vi "LS One Hour Data Loop.vi"(11 "FPGA OneHour Ref":T1) -> ()   [LabVIEW 2013]
uses:
  Controls/FPGA_OneHour_Reference.ctl
  <vilib>/rvi/interface/common/niFpgaWaitOnOcc.vi
  <vilib>/Utility/error.llb/Error Cluster From Error Code.vi
  <vilib>/rvi/errors/niLvFpgaAdjustHostInterfaceError.vi
  <vilib>/rvi/interface/nirviMethod/nirviMethod.xnode
  FPGA Bitfiles/LSDurabilityMain_Alternate.lvbitx
  <vilib>/rvi/interface/nirviReadWriteControl/nirviReadWriteControl.xnode
  <vilib>/FPGAPlugInAG/sbRIO-9626/niLvFpga_ReadFifo_sbRIO-9626.vi
  <vilib>/rvi/errors/niLvFpgaMergeErrorWithErrorCode.vi
  NiFpgaLv.dll
panel:
  in  "LoopWait(ms)":u32=100
  in  "Sections":i32=100
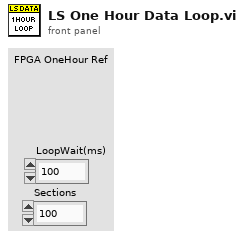
[diagram p1: front panel]
types:
  T1 = typedef "FPGA_OneHour_Reference.ctl" = refnum<k20>
  T2 = cluster{"FPGA OneHour Ref":T1, "Time":dbl, "PtsTaken":i32, "Pts/File":i32, "10AveWait":u32, "Stored Filepath":path, "FileIndex":i32, "FilesUsed":i32}
  T3 = enum16{"open", "replace", "create", "open or create", "replace or create", "replace or create with confirmation"}
  T4 = cluster{"Running?":bool, "Profile Record":bool, "RecordInterval":i32, "RecordDuration":i32, "RecordFreq":i32, "Data Filepath":path, "Hr Record":bool, "Serial Numbers":string[]}
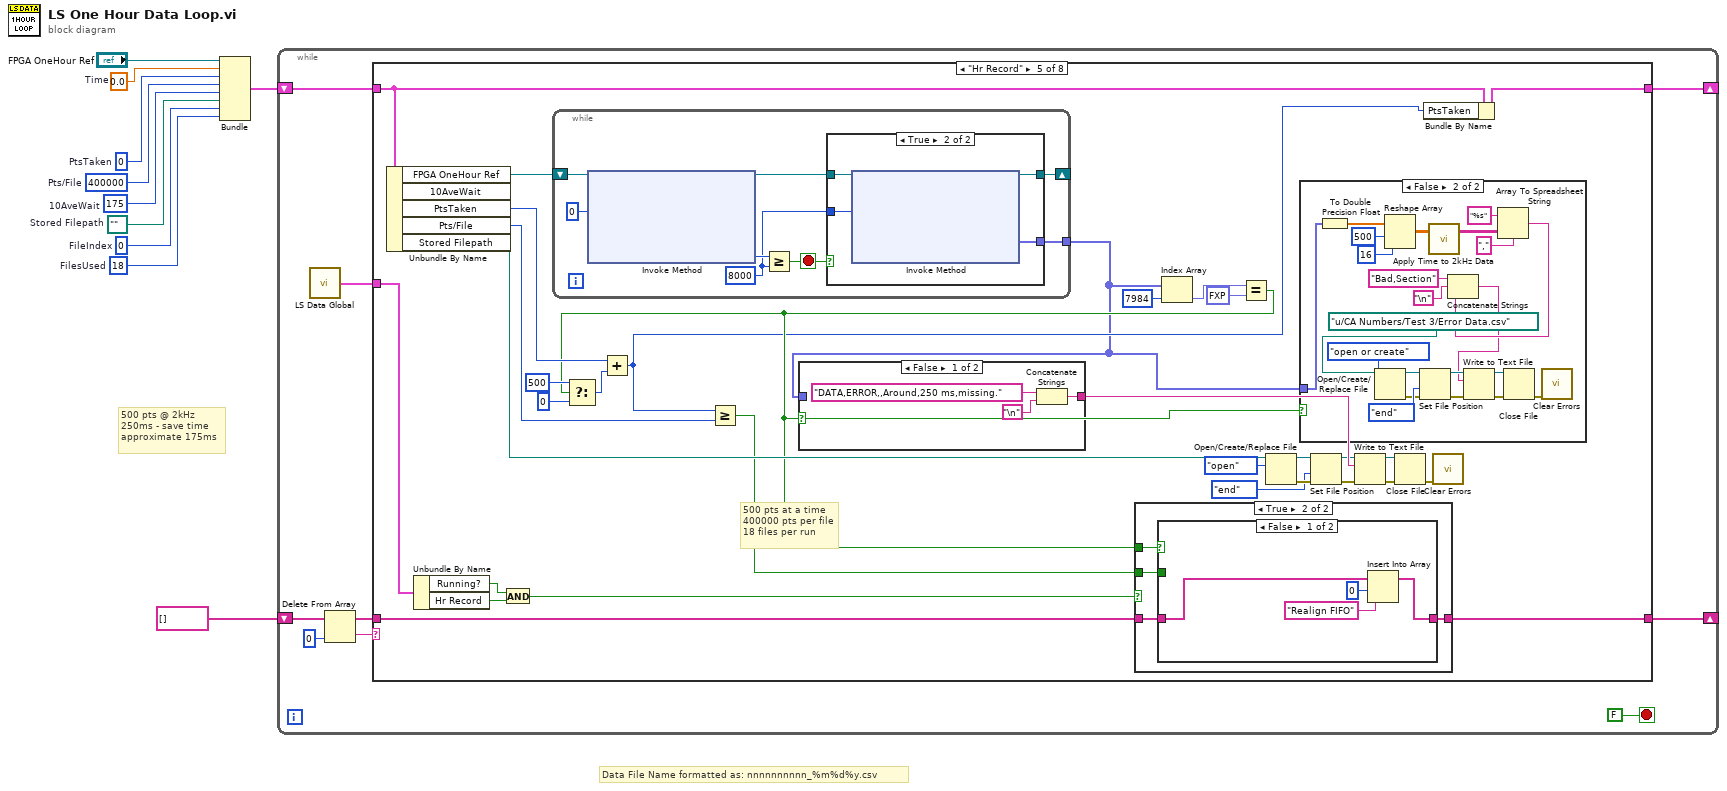
[diagram p0: block diagram]
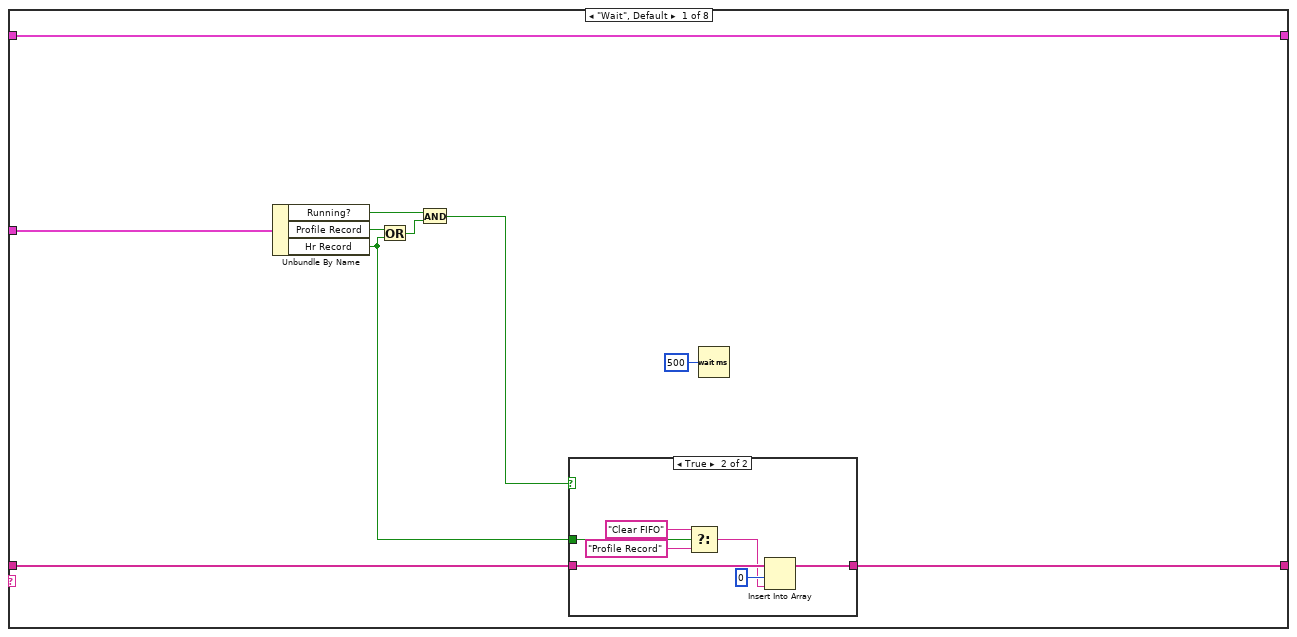
[diagram p2: hidden frame]
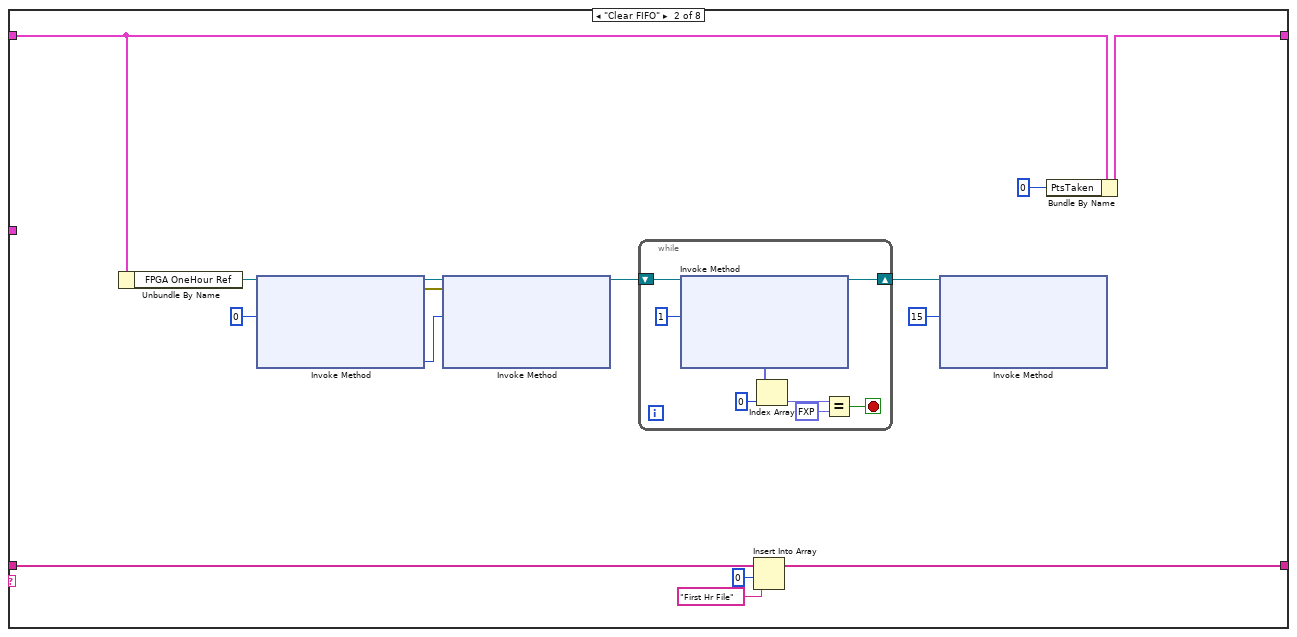
[diagram p4: hidden frame]
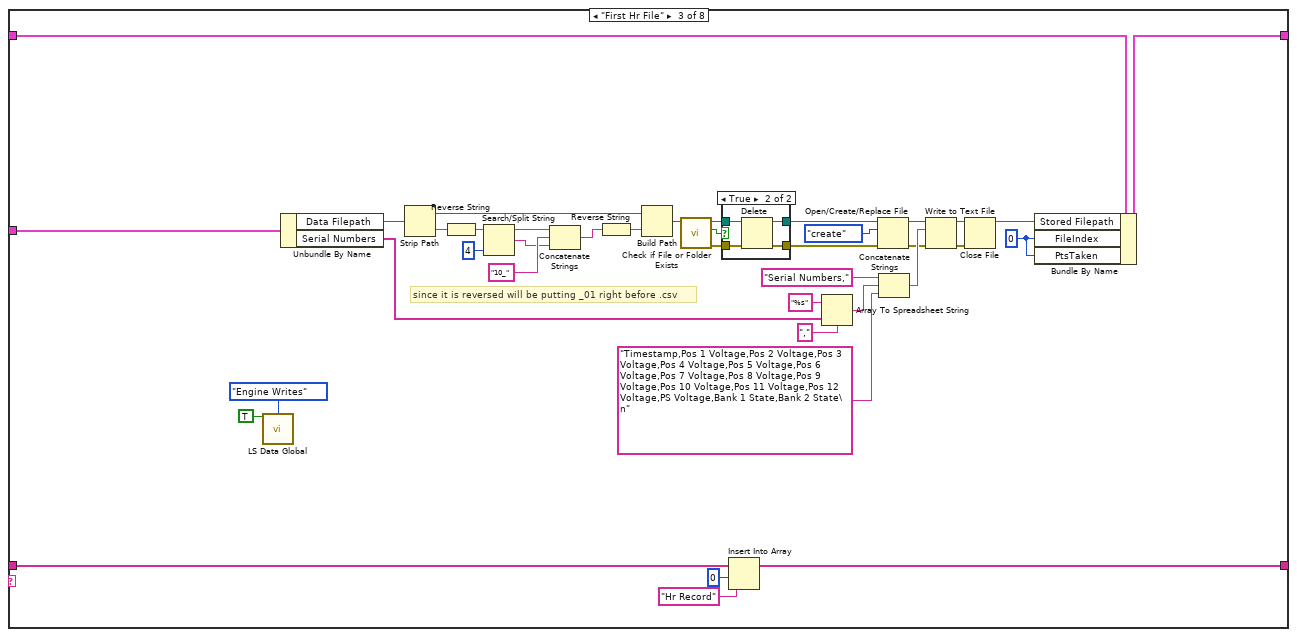
[diagram p5: hidden frame]
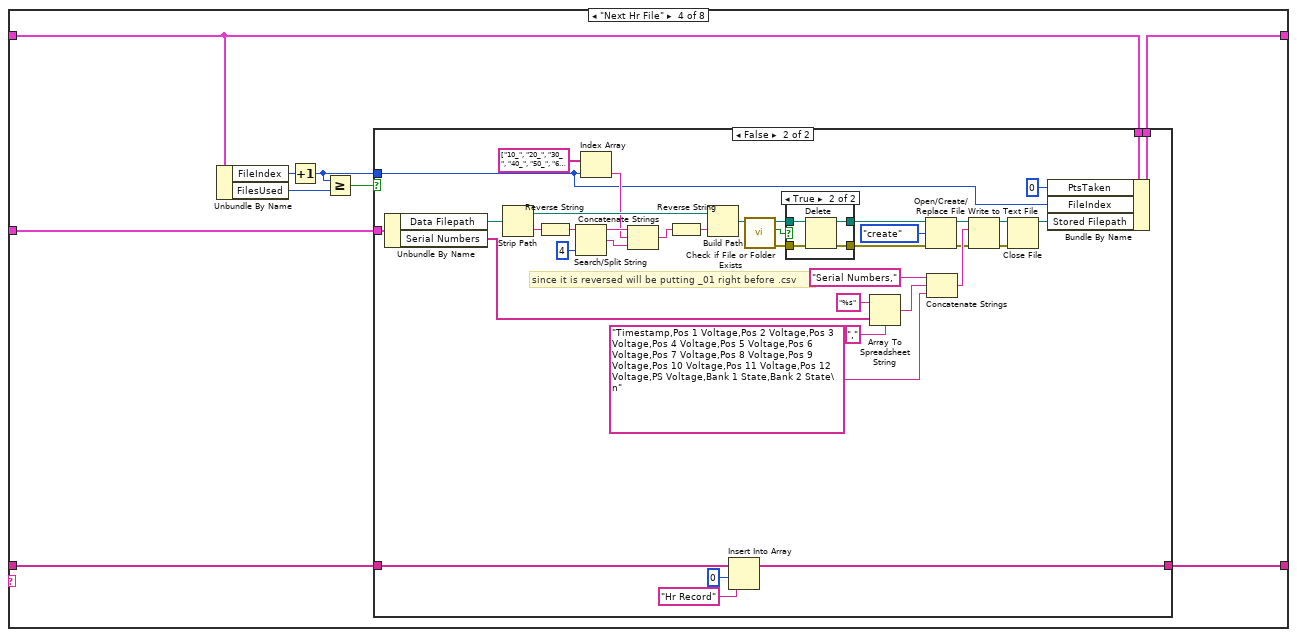
[diagram p7: hidden frame]
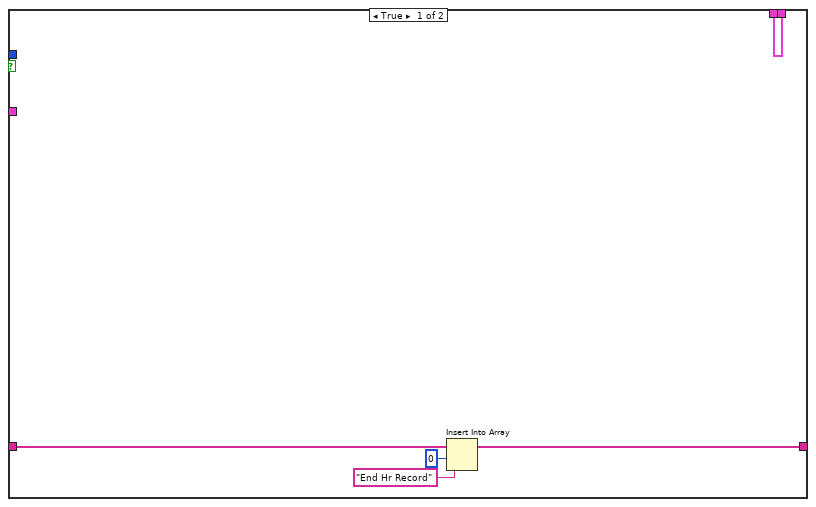
[diagram p8: hidden frame]
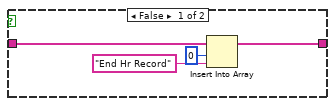
[diagram p11: hidden frame]
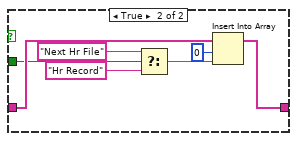
[diagram p12: hidden frame]
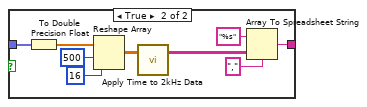
[diagram p13: hidden frame]
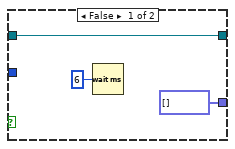
[diagram p14: hidden frame]
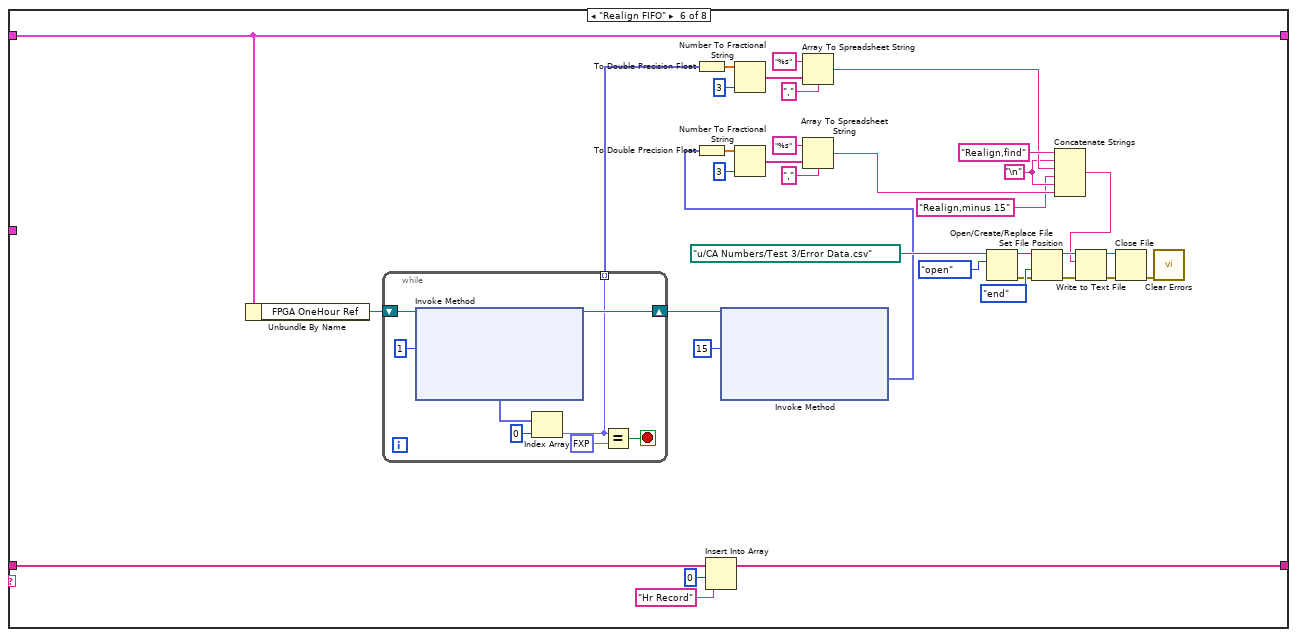
[diagram p15: hidden frame]
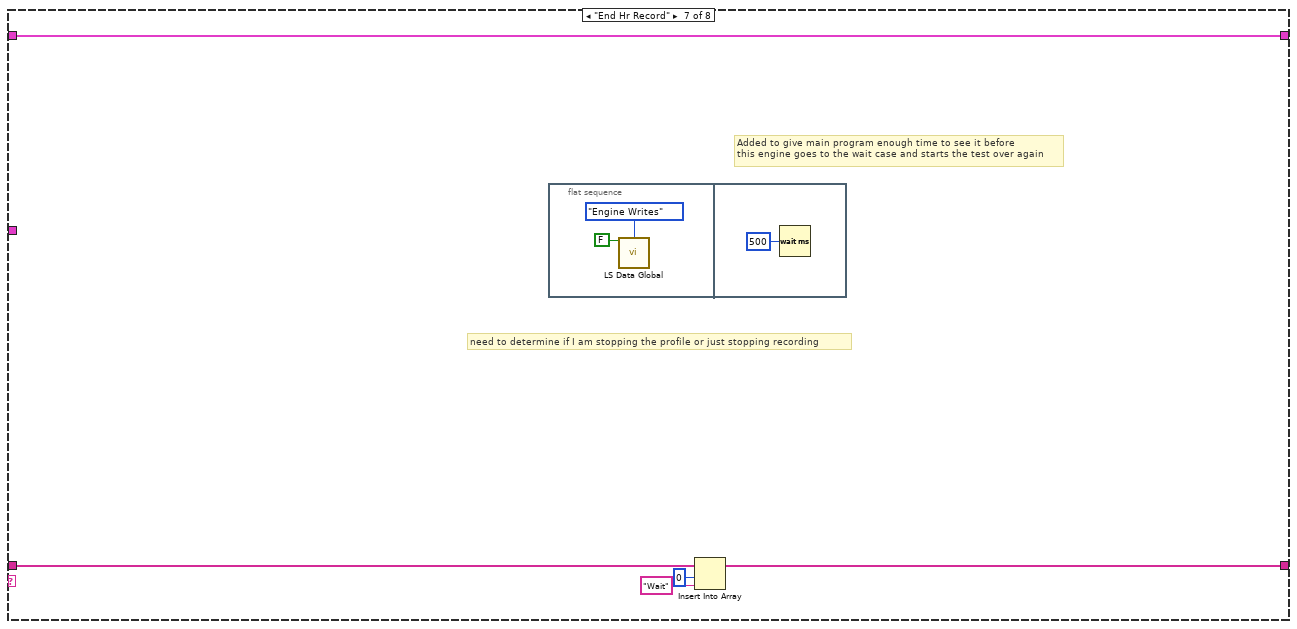
[diagram p16: hidden frame]
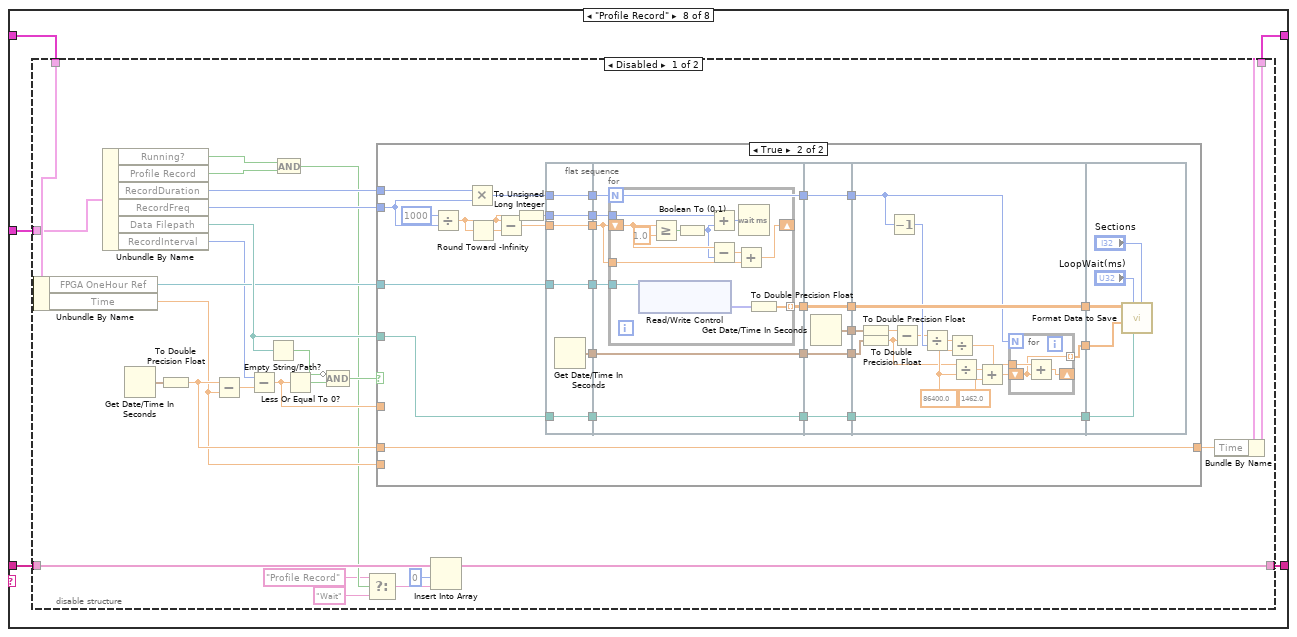
[diagram p17: hidden frame]
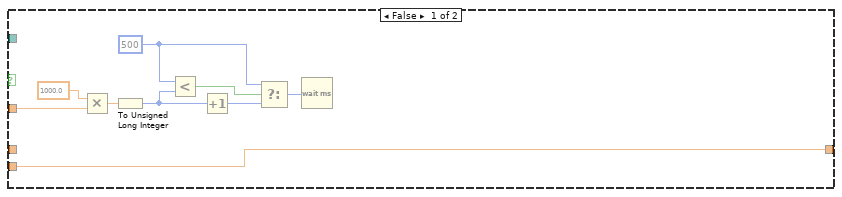
[diagram p18: hidden frame]
diagram:
  w1 = 18  # FilesUsed
  w2 = 400000  # Pts/File
  w4 = 0  # FileIndex
  w5 = path ""  # Stored Filepath
  w6 = u32 175  # 10AveWait
  w7 = 0  # PtsTaken
  w10 = 0.0  # Time
  # "500 pts @ 2kHz\n250ms - save time\napproximate 175ms"
  # "Data File Name formatted as: nnnnnnnnnn_%m%d%y.csv"
  n1 = Bundle("FPGA OneHour Ref"="FPGA OneHour Ref", "Time"=w10, "PtsTaken"=w7, "Pts/File"=w2, "10AveWait"=w6, "Stored Filepath"=w5, "FileIndex"=w4, "FilesUsed"=w1) -> (w9:T2)  [unwired: 1 in]
  n2 = while {
    shift-right: [w17] -> _
    shift-left: w9 -> [w18]
    shift-right: [w14] -> _
    shift-left: string[] [] -> [w16]
    stop <- FALSE stop-if-true
    n3 = call "LS Data Global.vi"() -> ("LS Cluster Out"=w15:T4)  [unwired: 14 in, 1 out]
    n4 = Delete From Array(array=w16, index=0) -> (deleted portion=w12:string, array with subset deleted=w11:string[])  [unwired: 1 in]
    n5 = case shown="\"Hr Record\"" w12 {
      tunnel: w11 -> [w26 w47 w86 w106 w177 w294 w312 w318]
      tunnel: [w25 w45 w85 w112 w178 w293 w311 w317] -> w14
      tunnel: w15 -> [w27 _ w98 w114 w194 _ _ w319]
      tunnel: w18 -> [w24 w43 w99 w111 w172 w297 w313 w321]
      tunnel: [w24 w42 w97 w113 w171 w297 w313 w320] -> w17
      frame "Wait", Default {
        n6 = Unbundle By Name(w27) -> ("Running?"=w28:bool, "Profile Record"=w23:bool, "Hr Record"=w21:bool)
        n7 = Or(x=w23, y=w21) -> (x .or. y?=w22:bool)
        n8 = And(x=w28, y=w22) -> (x .and. y?=w20:bool)
        n9 = case shown="True" w20 {
          tunnel: w26 -> [w30 w37]
          tunnel: [w30 w36] -> w25
          tunnel: w21 -> [_ w34]
          frame False {
          }
          frame True {
            n10 = Select(t="Clear FIFO" ("new element/subarray"), s=w34, f="Profile Record" ("new element/subarray")) -> (s? t:f=w32:string)
            n11 = Insert Into Array(array=w37, index=0, new element=w32) -> (w36:string[])
          }
        }
        n12 = Wait (ms)(milliseconds to wait=u32 500) -> ()  [unwired: 1 out]
      }
      frame "Clear FIFO" {
        n13 = Unbundle By Name(w43) -> ("FPGA OneHour Ref"=w52:T1)
        n14 = xnode "Invoke Method"("FPGA VI Reference In"=w52, "Number of Elements"=u32 0) -> ("FPGA VI Reference Out"=w51:T1, "error out"=w50:errorcluster, "Elements Remaining"=w48:u32)  [unwired: 2 in, 1 out]
        n15 = xnode "Invoke Method"("FPGA VI Reference In"=w51, "error in"=w50, "Number of Elements"=w48) -> ("FPGA VI Reference Out"=w40:T1)  [unwired: 1 in, 3 out]
        n16 = while {
          shift-right: [w59] -> w38
          shift-left: w40 -> [w60]
          stop <- w53 stop-if-true
          n17 = xnode "Invoke Method"("FPGA VI Reference In"=w60, "Number of Elements"=u32 1) -> ("FPGA VI Reference Out"=w59:T1, "Data"=w57:fxp<+/-,18,5>[])  [unwired: 2 in, 2 out]
          n18 = Index Array(array=w57, index=0) -> (element=w55:fxp<+/-,18,5>)
          n19 = Equal?(x=w55, y=fxp<+/-,18,5> -15.0 ("lower limit")) -> (x = y?=w53:bool)
        }
        n20 = Insert Into Array(array=w47, index=0, new element="First Hr File" ("new element/subarray")) -> (w45:string[])
        n21 = xnode "Invoke Method"("FPGA VI Reference In"=w38, "Number of Elements"=u32 15) -> ()  [unwired: 2 in, 4 out]
        n22 = Bundle By Name(cluster=w43, "PtsTaken"=0) -> (w42:T2)
      }
      frame "First Hr File" {
        w63 = 0 ("FileIndex")
        # "since it is reversed will be putting _01 right before .csv"
        n23 = call "LS Data Global.vi"("Recording In"=TRUE, "Mode"=enum16{"Read", "Engine Writes", "Main Writes"}."Engine Writes") -> ()  [unwired: 12 in, 2 out]
        n24 = Unbundle By Name(w98) -> ("Data Filepath"=w96:path, "Serial Numbers"=w64:string[])
        n25 = Strip Path(path=w96) -> (stripped path=w95:path, name=w94:string)
        n26 = Reverse String(1:w94) -> (0:w92:string)
        n27 = Search/Split String(string=w92, offset (0)=4) -> (substring before match=w90:string, match + rest of string=w87:string)  [unwired: 1 in, 1 out]
        n28 = Concatenate Strings(w90, "10_", w87) -> (w89:string)
        n29 = Reverse String(1:w89) -> (0:w93:string)
        n30 = Build Path(base path=w95, name or relative path=w93) -> (appended path=w82:path)
        n31 = call <vilib>:"Check if File or Folder Exists.vi"("path"=w82) -> ("error out"=w67:errorcluster, "file or folder exists?"=w81:bool, "dup path"=w80:path)  [unwired: 8 in]
        n32 = case shown="True" w81 {
          tunnel: w80 -> [w101 w105]
          tunnel: [w101 w104] -> w69
          tunnel: w67 -> [w100 w103]
          tunnel: [w100 w102] -> w66
          frame False {
          }
          frame True {
            n33 = Delete(path (use dialog)=w105, error in=w103) -> (deleted path=w104:path, error out=w102:errorcluster)  [unwired: 3 in, 1 out]
          }
        }
        n34 = Insert Into Array(array=w86, index=0, new element="Hr Record" ("new element/subarray")) -> (w85:string[])
        n35 = Array To Spreadsheet String(delimiter (Tab)=",", array=w64, 3:"%s" ("format string")) -> (spreadsheet string=w79:string)
        n36 = Open/Create/Replace File(file path (use dialog)=w69, error in=w66, operation (0:open)=T3."create") -> (refnum out=w73:refnum<file>, error out=w71:errorcluster)  [unwired: 3 in, 1 out]
        n37 = Concatenate Strings("Serial Numbers," ("string"), w79, "Timestamp,Pos 1 Voltage,Pos 2 Voltage,Pos 3 Voltage,Pos 4 Voltage,Pos 5 Voltage,Pos 6 Voltage,Pos 7 Voltage,Pos 8 Voltage,Pos 9 Voltage,Pos 10 Voltage,Pos 11 Voltage,Pos 12 Voltage,PS Voltage,Bank 1 State,Bank 2 State\n") -> (w76:string)
        n38 = Write to Text File(file (use dialog)=w73, text=w76, error in=w71) -> (refnum out=w74:refnum<file>, error out=w72:errorcluster)  [unwired: 1 in, 1 out]
        n39 = Close File(refnum=w74, error in=w72) -> (path=w68:path)  [unwired: 1 out]
        n40 = Bundle By Name(cluster=w99, "Stored Filepath"=w68, "FileIndex"=w63, "PtsTaken"=w63) -> (w97:T2)
      }
      frame "Next Hr File" {
        n41 = Unbundle By Name(w111) -> ("FileIndex"=w110:i32, "FilesUsed"=w109:i32)
        n42 = Increment(x=w110) -> (x+1=w108:i32)
        n43 = Greater Or Equal?(x=w108, y=w109) -> (x >= y?=w107:bool)
        n44 = case shown="False" w107 {
          tunnel: w114 -> [_ w158]
          tunnel: [w119 w157] -> w113
          tunnel: [w117 w146] -> w112
          tunnel: w111 -> [w119 w124]
          tunnel: w108 -> [_ w121]
          tunnel: w106 -> [w118 w147]
          frame True {
            n45 = Insert Into Array(array=w118, index=0, new element="End Hr Record" ("new element/subarray")) -> (w117:string[])
          }
          frame False {
            # "since it is reversed will be putting _01 right before .csv"
            n46 = Unbundle By Name(w158) -> ("Data Filepath"=w156:path, "Serial Numbers"=w125:string[])
            n47 = Strip Path(path=w156) -> (stripped path=w155:path, name=w154:string)
            n48 = Reverse String(1:w154) -> (0:w152:string)
            n49 = Search/Split String(string=w152, offset (0)=4) -> (substring before match=w150:string, match + rest of string=w148:string)  [unwired: 1 in, 1 out]
            n50 = Index Array(array=string[] ["10_", "20_", "30_", "40_", "50_", "60_", "70_", "80_", "90_", "01_", "11_", "21_", "31_", "41_", "51_", "61_", "71_", "81_", "91_", "02_", "12_", "22_", "32_", "42_", "52_", "62_", "72_", "82_", "92_", "03_", "13_", "23_"], index=w121) -> (element=w122:string)
            n51 = Concatenate Strings(w150, w122, w148) -> (w149:string)
            n52 = Reverse String(1:w149) -> (0:w153:string)
            n53 = Build Path(base path=w155, name or relative path=w153) -> (appended path=w143:path)
            n54 = Insert Into Array(array=w147, index=0, new element="Hr Record" ("new element/subarray")) -> (w146:string[])
            n55 = call <vilib>:"Check if File or Folder Exists.vi"("path"=w143) -> ("error out"=w128:errorcluster, "file or folder exists?"=w142:bool, "dup path"=w141:path)  [unwired: 8 in]
            n56 = case shown="True" w142 {
              tunnel: w141 -> [w160 w164]
              tunnel: [w160 w163] -> w130
              tunnel: w128 -> [w159 w162]
              tunnel: [w159 w161] -> w127
              frame False {
              }
              frame True {
                n57 = Delete(path (use dialog)=w164, error in=w162) -> (deleted path=w163:path, error out=w161:errorcluster)  [unwired: 3 in, 1 out]
              }
            }
            n58 = Array To Spreadsheet String(delimiter (Tab)=",", array=w125, 3:"%s" ("format string")) -> (spreadsheet string=w140:string)
            n59 = Open/Create/Replace File(file path (use dialog)=w130, error in=w127, operation (0:open)=T3."create") -> (refnum out=w134:refnum<file>, error out=w132:errorcluster)  [unwired: 3 in, 1 out]
            n60 = Concatenate Strings("Serial Numbers," ("string"), w140, "Timestamp,Pos 1 Voltage,Pos 2 Voltage,Pos 3 Voltage,Pos 4 Voltage,Pos 5 Voltage,Pos 6 Voltage,Pos 7 Voltage,Pos 8 Voltage,Pos 9 Voltage,Pos 10 Voltage,Pos 11 Voltage,Pos 12 Voltage,PS Voltage,Bank 1 State,Bank 2 State\n") -> (w137:string)
            n61 = Write to Text File(file (use dialog)=w134, text=w137, error in=w132) -> (refnum out=w135:refnum<file>, error out=w133:errorcluster)  [unwired: 1 in, 1 out]
            n62 = Close File(refnum=w135, error in=w133) -> (path=w129:path)  [unwired: 1 out]
            n63 = Bundle By Name(cluster=w124, "PtsTaken"=0, "FileIndex"=w121, "Stored Filepath"=w129) -> (w157:T2)
          }
        }
      }
      frame "Hr Record" {
        # "500 pts at a time\n400000 pts per file\n18 files per run"
        n64 = Unbundle By Name(w172) -> ("FPGA OneHour Ref"=w166:T1, "PtsTaken"=w176:i32, "Pts/File"=w170:i32, "Stored Filepath"=w183:path)  [unwired: 1 out]
        n65 = Unbundle By Name(w194) -> ("Running?"=w195:bool, "Hr Record"=w196:bool)
        n66 = And(x=w195, y=w196) -> (x .and. y?=w179:bool)
        n67 = while {
          shift-right: [w252] -> _
          shift-left: w166 -> [w255]
          tunnel: [w251] -> w165
          stop <- w250 stop-if-true
          w254 = u32 8000 ("y")
          n68 = xnode "Invoke Method"("FPGA VI Reference In"=w255, "Number of Elements"=u32 0) -> ("FPGA VI Reference Out"=w253:T1, "Elements Remaining"=w256:u32)  [unwired: 2 in, 2 out]
          n69 = Greater Or Equal?(x=w256, y=w254) -> (x >= y?=w250:bool)
          n70 = case shown="True" w250 {
            tunnel: w254 -> [_ w264]
            tunnel: w253 -> [w260 w263]
            tunnel: [w260 w262] -> w252
            tunnel: [fxp<+/-,18,5>[] [] ("Data") w261] -> w251
            frame False {
              n71 = Wait (ms)(milliseconds to wait=u32 6) -> ()  [unwired: 1 out]
            }
            frame True {
              n72 = xnode "Invoke Method"("FPGA VI Reference In"=w263, "Number of Elements"=w264) -> ("FPGA VI Reference Out"=w262:T1, "Data"=w261:fxp<+/-,18,5>[])  [unwired: 2 in, 2 out]
            }
          }
        }
        n73 = Index Array(array=w165, index=7984) -> (element=w181:fxp<+/-,18,5>)
        n74 = Equal?(x=w181, y=fxp<+/-,18,5> -15.0) -> (x = y?=w168:bool)
        n75 = Select(t=500 ("PtsTaken"), s=w168, f=0 ("PtsTaken")) -> (s? t:f=w173:i32)
        n76 = Add(x=w176, y=w173) -> (x+y=w167:i32)
        n77 = Greater Or Equal?(x=w167, y=w170) -> (x >= y?=w169:bool)
        n78 = case shown="False" w168 {
          tunnel: [w238 w244] -> w186
          tunnel: w165 -> [_ w243]
          frame False {
            n79 = Concatenate Strings("DATA,ERROR,,Around,250 ms,missing." ("string"), "\n") -> (w238:string)
          }
          frame True {
            n80 = To Double Precision Float(number=w243) -> (double precision float=w247:dbl[])
            n81 = Reshape Array(w247, 500 ("dimension size"), 16 ("dimension size")) -> (w242:dbl[][])
            n82 = call "Apply Time to 2kHz Data.vi"("Data In"=w242) -> ("Data Out"=w241:string[][])  [unwired: 2 in]
            n83 = Array To Spreadsheet String(delimiter (Tab)=",", array=w241, 3:"%s" ("format string")) -> (spreadsheet string=w244:string)
          }
        }
        n84 = case shown="True" w179 {
          tunnel: w177 -> [w221 w225]
          tunnel: [w220 w224] -> w178
          tunnel: w168 -> [_ w226]
          tunnel: w169 -> [_ w223]
          frame False {
            n85 = Insert Into Array(array=w221, index=0, new element="End Hr Record") -> (w220:string[])
          }
          frame True {
            n86 = case shown="False" w226 {
              tunnel: w225 -> [w230 w237]
              tunnel: [w229 w236] -> w224
              tunnel: w223 -> [_ w234]
              frame False {
                n87 = Insert Into Array(array=w230, index=0, new element="Realign FIFO" ("new element/subarray")) -> (w229:string[])
              }
              frame True {
                n88 = Select(t="Next Hr File", s=w234, f="Hr Record") -> (s? t:f=w233:string)
                n89 = Insert Into Array(array=w237, index=0, new element=w233) -> (w236:string[])
              }
            }
          }
        }
        n90 = Open/Create/Replace File(file path (use dialog)=w183, operation (0:open)=T3."open") -> (refnum out=w189:refnum<file>, error out=w188:errorcluster)  [unwired: 4 in, 1 out]
        n91 = case shown="False" w168 {
          tunnel: w165 -> [_ w213]
          frame True {
          }
          frame False {
            n92 = To Double Precision Float(number=w213) -> (double precision float=w216:dbl[])
            n93 = Open/Create/Replace File(file path (use dialog)=path "u:/CA Numbers/Test 3/Error Data.csv" ("base path"), operation (0:open)=T3."open or create") -> (refnum out=w206:refnum<file>, error out=w207:errorcluster)  [unwired: 4 in, 1 out]
            n94 = Reshape Array(w216, 500 ("dimension size"), 16 ("dimension size")) -> (w212:dbl[][])
            n95 = Set File Position(refnum=w206, from (0:start)=enum16{"start", "end", "current"}."end", error in=w207) -> (refnum out=w209:refnum<file>, error out=w210:errorcluster)  [unwired: 1 in]
            n96 = call "Apply Time to 2kHz Data.vi"("Data In"=w212) -> ("Data Out"=w211:string[][])  [unwired: 2 in]
            n97 = Array To Spreadsheet String(delimiter (Tab)=",", array=w211, 3:"%s" ("format string")) -> (spreadsheet string=w199:string)
            n98 = Concatenate Strings("Bad,Section" ("string"), "\n", w199) -> (w198:string)
            n99 = Write to Text File(file (use dialog)=w209, text=w198, error in=w210) -> (refnum out=w203:refnum<file>, error out=w202:errorcluster)  [unwired: 1 in, 1 out]
            n100 = Close File(refnum=w203, error in=w202) -> (error out=w204:errorcluster)  [unwired: 1 out]
            n101 = call <vilib>:"Clear Errors.vi"("error in (no error)"=w204) -> ()  [unwired: 6 in, 1 out]
          }
        }
        n102 = Set File Position(refnum=w189, from (0:start)=enum16{"start", "end", "current"}."end", error in=w188) -> (refnum out=w185:refnum<file>, error out=w184:errorcluster)  [unwired: 1 in]
        n103 = Write to Text File(file (use dialog)=w185, text=w186, error in=w184) -> (refnum out=w192:refnum<file>, error out=w193:errorcluster)  [unwired: 1 in, 1 out]
        n104 = Close File(refnum=w192, error in=w193) -> (error out=w191:errorcluster)  [unwired: 1 out]
        n105 = Bundle By Name(cluster=w172, "PtsTaken"=w167) -> (w171:T2)
        n106 = call <vilib>:"Clear Errors.vi"("error in (no error)"=w191) -> ()  [unwired: 6 in, 1 out]
      }
      frame "Realign FIFO" {
        w273 = "\n"
        n107 = Unbundle By Name(w297) -> ("FPGA OneHour Ref"=w300:T1)
        n108 = while {
          shift-right: [w307] -> w298
          shift-left: w300 -> [w308]
          tunnel: [w301] -> w277 mode=indexing
          stop <- w302 stop-if-true
          n109 = xnode "Invoke Method"("FPGA VI Reference In"=w308, "Number of Elements"=u32 1) -> ("FPGA VI Reference Out"=w307:T1, "Data"=w305:fxp<+/-,18,5>[])  [unwired: 2 in, 2 out]
          n110 = Index Array(array=w305, index=0) -> (element=w301:fxp<+/-,18,5>)
          n111 = Equal?(x=w301, y=fxp<+/-,18,5> -15.0 ("lower limit")) -> (x = y?=w302:bool)
        }
        n112 = To Double Precision Float(number=w277) -> (double precision float=w275:dbl[])
        n113 = Insert Into Array(array=w294, index=0, new element="Hr Record" ("new element/subarray")) -> (w293:string[])
        n114 = xnode "Invoke Method"("FPGA VI Reference In"=w298, "Number of Elements"=u32 15) -> ("Data"=w267:fxp<+/-,18,5>[])  [unwired: 2 in, 3 out]
        n115 = To Double Precision Float(number=w267) -> (double precision float=w271:dbl[])
        n116 = Number To Fractional String(number=w275, precision (6)=i16 3) -> (F-format string=w274:string[])  [unwired: 2 in]
        n117 = Number To Fractional String(number=w271, precision (6)=i16 3) -> (F-format string=w272:string[])  [unwired: 2 in]
        n118 = Array To Spreadsheet String(delimiter (Tab)=",", array=w274, 3:"%s" ("format string")) -> (spreadsheet string=w280:string)
        n119 = Array To Spreadsheet String(delimiter (Tab)=",", array=w272, 3:"%s" ("format string")) -> (spreadsheet string=w266:string)
        n120 = Open/Create/Replace File(file path (use dialog)=path "u:/CA Numbers/Test 3/Error Data.csv" ("base path"), operation (0:open)=T3."open") -> (refnum out=w286:refnum<file>, error out=w287:errorcluster)  [unwired: 4 in, 1 out]
        n121 = Set File Position(refnum=w286, from (0:start)=enum16{"start", "end", "current"}."end", error in=w287) -> (refnum out=w289:refnum<file>, error out=w290:errorcluster)  [unwired: 1 in]
        n122 = Concatenate Strings("Realign,find" ("string"), w273, w280, "Realign,minus 15" ("string"), w273, w266) -> (w279:string)
        n123 = Write to Text File(file (use dialog)=w289, text=w279, error in=w290) -> (refnum out=w283:refnum<file>, error out=w282:errorcluster)  [unwired: 1 in, 1 out]
        n124 = Close File(refnum=w283, error in=w282) -> (error out=w284:errorcluster)  [unwired: 1 out]
        n125 = call <vilib>:"Clear Errors.vi"("error in (no error)"=w284) -> ()  [unwired: 6 in, 1 out]
      }
      frame "End Hr Record" {
        # "Added to give main program enough time to see it before\nthis engine goes to the wait case and starts the test over again"
        # "need to determine if I am stopping the profile or just stopping recording"
        n126 = flat-sequence {
          frame #0 {
            n127 = call "LS Data Global.vi"("Recording In"=FALSE, "Mode"=enum16{"Read", "Engine Writes", "Main Writes"}."Engine Writes") -> ()  [unwired: 12 in, 2 out]
          }
          frame #1 {
            n128 = Wait (ms)(milliseconds to wait=u32 500) -> ()  [unwired: 1 out]
          }
        }
        n129 = Insert Into Array(array=w312, index=0, new element="Wait" ("new element/subarray")) -> (w311:string[])
      }
      frame "Profile Record" {
        n130 = disable-structure shown="Disabled" {
          disable-tunnel: w321 -> [w347 w441]
          disable-tunnel: [w346 w441] -> w320
          disable-tunnel: w319 -> [w345 _]
          disable-tunnel: w318 -> [w328 w440]
          disable-tunnel: [w327 w440] -> w317
          frame Disabled {
            n131 = Unbundle By Name(w347) -> ("FPGA OneHour Ref"=w339:T1, "Time"=w333:dbl)
            n132 = Unbundle By Name(w345) -> ("Running?"=w330:bool, "Profile Record"=w329:bool, "RecordDuration"=w342:i32, "RecordFreq"=w343:i32, "Data Filepath"=w344:path, "RecordInterval"=w331:i32)
            n133 = Get Date/Time In Seconds() -> (seconds since 1Jan1904=w341:timestamp)
            n134 = To Double Precision Float(number=w341) -> (double precision float=w334:dbl)
            n135 = Subtract(x=w334, y=w333) -> (x-y=w338:dbl)
            n136 = Subtract(x=w331, y=w338) -> (x-y=w332:dbl)
            n137 = Empty String/Path?(string/path=w344) -> (empty?=w336:bool)
            n138 = And(x=w330, y=w329) -> (x .and. y?=w325:bool)
            n139 = Less Or Equal To 0?(x=w332) -> (x <= 0?=w337:bool)
            n140 = Compound Arithmetic op=AND(invert w336, w337) -> (w335:bool)
            n141 = Select(t="Profile Record", s=w325, f="Wait") -> (s? t:f=w322:string)
            n142 = case shown="True" w335 {
              tunnel: w343 -> [_ w378]
              tunnel: w342 -> [_ w384]
              tunnel: w339 -> [_ w381]
              tunnel: w334 -> [_ w380]
              tunnel: [w356 w380] -> w340
              tunnel: w333 -> [w356 _]
              tunnel: w332 -> [w350 _]
              tunnel: w344 -> [_ w357]
              frame False {
                w355 = u32 500 ("milliseconds to wait")
                n143 = Multiply(x=1000.0 ("y"), y=w350) -> (x*y=w352:dbl)
                n144 = To Unsigned Long Integer(number=w352) -> (unsigned 32bit integer=w349:u32)
                n145 = Less?(x=w355, y=w349) -> (x < y?=w353:bool)
                n146 = Increment(x=w349) -> (x+1=w348:u32)
                n147 = Select(t=w355, s=w353, f=w348) -> (s? t:f=w354:u32)
                n148 = Wait (ms)(milliseconds to wait=w354) -> ()  [unwired: 1 out]
              }
              frame True {
                n149 = Divide(x=1000, y=w378) -> (x/y=w383:dbl)
                n150 = Multiply(x=w384, y=w378) -> (x*y=w371:i32)
                n151 = Round Toward -Infinity(1:w383) -> (0:w385:dbl)
                n152 = Subtract(x=w383, y=w385) -> (x-y=w377:dbl)
                n153 = To Unsigned Long Integer(number=w383) -> (unsigned 32bit integer=w382:u32)
                n154 = flat-sequence {
                  tunnel: w377 -> [w388]
                  tunnel: w381 -> [w389]
                  tunnel: w382 -> [w390]
                  tunnel: w371 -> [w391]
                  tunnel: [w391] -> w376
                  tunnel: [w390] -> w375
                  tunnel: [w389] -> w374
                  tunnel: [w388] -> w373
                  tunnel: [w387] -> w366
                  tunnel: [w386] -> w358
                  tunnel: w357 -> [w386]
                  tunnel: w376 -> [w394]
                  tunnel: w375 -> [w398]
                  tunnel: w374 -> [w397]
                  tunnel: w373 -> [w392]
                  tunnel: [w396] -> w372
                  tunnel: [w395] -> w367
                  tunnel: w366 -> [w395]
                  tunnel: [w394] -> w364
                  tunnel: [w393] -> w359
                  tunnel: w358 -> [w393]
                  tunnel: w372 -> [w415]
                  tunnel: [w415] -> w370
                  tunnel: [w414] -> w369
                  tunnel: [w413] -> w368
                  tunnel: w367 -> [w413]
                  tunnel: [w412] -> w365
                  tunnel: w364 -> [w412]
                  tunnel: [w411] -> w360
                  tunnel: w359 -> [w411]
                  tunnel: w370 -> [w431]
                  tunnel: w369 -> [w425]
                  tunnel: w368 -> [w424]
                  tunnel: w365 -> [w423]
                  tunnel: [w431] -> w363
                  tunnel: [w421] -> w362
                  tunnel: [w418] -> w361
                  tunnel: w360 -> [w418]
                  tunnel: w361 -> [w437]
                  tunnel: w362 -> [w438]
                  tunnel: w363 -> [w439]
                  frame #0 {
                    n155 = Get Date/Time In Seconds() -> (seconds since 1Jan1904=w387:timestamp)
                  }
                  frame #1 {
                    n156 = for {
                      N: w394 -> [_]
                      tunnel: w398 -> [w410]
                      shift-right: [w407] -> _
                      shift-left: w392 -> [w408]
                      tunnel: w392 -> [w406]
                      tunnel: w397 -> [w405]
                      tunnel: [w403] -> w396 mode=indexing
                      n157 = xnode "Read/Write Control"("FPGA VI Reference In"=w405) -> ("Analog Inputs"=w404:fxp<+/-,28,17>[])  [unwired: 1 in, 2 out]
                      n158 = Greater Or Equal?(x=w408, y=1.0) -> (x >= y?=w401:bool)
                      n159 = Boolean To (0,1)(Boolean=w401) -> (0, 1=w400:i16)
                      n160 = Add(x=w410, y=w400) -> (x+y=w409:u32)
                      n161 = Subtract(x=w408, y=w400) -> (x-y=w399:dbl)
                      n162 = Add(x=w399, y=w406) -> (x+y=w407:dbl)
                      n163 = Wait (ms)(milliseconds to wait=w409) -> ()  [unwired: 1 out]
                      n164 = To Double Precision Float(number=w404) -> (double precision float=w403:dbl[])
                    }
                  }
                  frame #2 {
                    n165 = Get Date/Time In Seconds() -> (seconds since 1Jan1904=w414:timestamp)
                  }
                  frame #3 {
                    w420 = 86400.0 ("y")
                    n166 = To Double Precision Float(number=w425) -> (double precision float=w419:dbl)
                    n167 = To Double Precision Float(number=w424) -> (double precision float=w416:dbl)
                    n168 = Decrement(x=w423) -> (x-1=w422:i32)
                    n169 = Subtract(x=w419, y=w416) -> (x-y=w417:dbl)
                    n170 = Divide(x=w417, y=w422) -> (x/y=w426:dbl)
                    n171 = Divide(x=w426, y=w420) -> (x/y=w430:dbl)
                    n172 = Divide(x=w416, y=w420) -> (x/y=w427:dbl)
                    n173 = Add(x=w427, y=1462.0) -> (x+y=w429:dbl)
                    n174 = for {
                      N: w423 -> [_]
                      shift-right: [w432] -> _
                      shift-left: w429 -> [w433]
                      tunnel: w430 -> [w434]
                      tunnel: [w433] -> w421 mode=indexing
                      n175 = Add(x=w434, y=w433) -> (x+y=w432:dbl)
                    }
                  }
                  frame #4 {
                    n176 = call "Format Data to Save.vi"("Sections"="Sections", "FilePath"=w437, "LoopBeginWait(ms)"="LoopWait(ms)", "Time"=w438, "Data"=w439) -> ()  [unwired: 7 in]
                  }
                }
              }
            }
            n177 = Insert Into Array(array=w328, index=0, new element=w322) -> (w327:string[])
            n178 = Bundle By Name(cluster=w347, "Time"=w340) -> (w346:T2)
          }
          frame Enabled {
          }
        }
      }
    }
  }
